vi "ClearAvailableRecord.vi"(8 "error in (no error)":errorcluster, 11 "FpgaRef5782 In":refnum<class "FpgaRefx410.lvclass">) -> (0 "error out":errorcluster, 3 "FpgaRef5782 Out":refnum<class "FpgaRefx410.lvclass">)   [LabVIEW 2025, in "FpgaRefx410.lvclass"]
uses:
  FpgaRefx410.lvclass
  FpgaRefx410.lvclass/FpgaRefx410.ctl
  <vilib>/Utility/error.llb/Error Cluster From Error Code.vi
  <vilib>/rvi/errors/niLvFpgaAdjustHostInterfaceError.vi
  <vilib>/rvi/interface/nirviMethod/nirviMethod.xnode
  x410 FPGA ref.ctl
  <vilib>/FPGAPlugInAG/Dynamic/niLvFpga_ReadFifo_Dynamic.vi
  <vilib>/rvi/errors/niLvFpgaMergeErrorWithErrorCode.vi
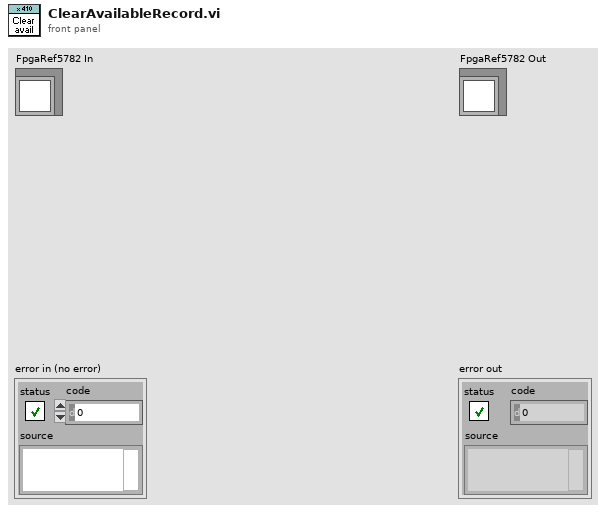
[diagram p1: front panel]
types:
  T1 = typedef "x410 FPGA ref.ctl" = refnum<k20>
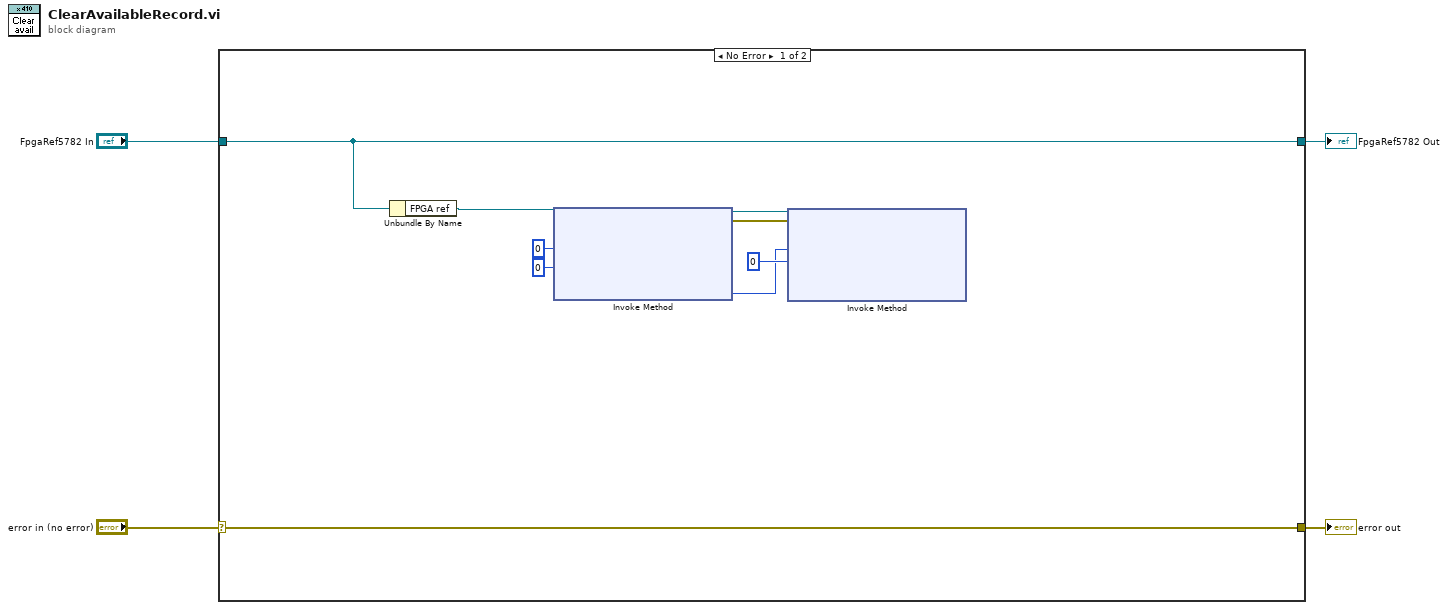
[diagram p0: block diagram]
diagram:
  n1 = case shown="No Error" "error in (no error)" {
    selector: "error in (no error)" -> [w13 w15]
    tunnel: [w13 w15] -> w3
    tunnel: [w12 w14] -> w1
    tunnel: "FpgaRef5782 In" -> [w12 w14]
    frame No Error {
      n2 = Unbundle By Name(w12) -> ("FPGA ref"=w5:T1)
      n3 = xnode "Invoke Method"("FPGA VI Reference In"=w5, "Number of Elements"=u32 0, "Timeout (ms)"=0) -> ("FPGA VI Reference Out"=w10:T1, "error out"=w11:errorcluster, "Elements Remaining"=w8:u32)  [unwired: 1 in, 1 out]
      n4 = xnode "Invoke Method"("FPGA VI Reference In"=w10, "error in"=w11, "Number of Elements"=w8, "Timeout (ms)"=0) -> ()  [unwired: 4 out]
    }
    frame Error {
    }
  }
  "error out" <- w3
  "FpgaRef5782 Out" <- w1
